vi "replace_file_extension.vi"(8 "error in (no error)":errorcluster, 10 "new_extension":string, 11 "data_path":path) -> (0 "error out":errorcluster, 3 "appended path":path)   [LabVIEW 2018]
panel:
  out "filename without extension":string
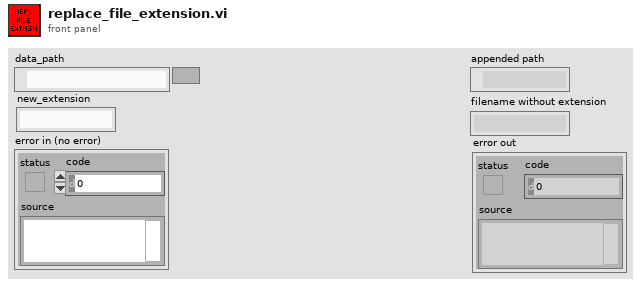
[diagram p1: front panel]
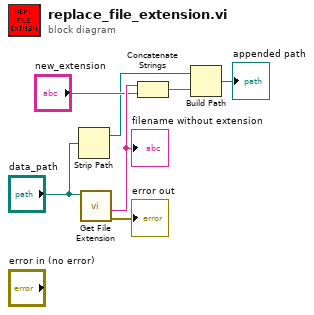
[diagram p0: block diagram]
diagram:
  n1 = Strip Path(path="data_path") -> (stripped path=w4:path)  [unwired: 1 out]
  n2 = call <vilib>:"Get File Extension.vi"("file"="data_path") -> ("error out"=→"error out":errorcluster, "filename without extension"=w7:string)  [unwired: 6 in, 3 out]
  "filename without extension" <- w7
  n3 = Concatenate Strings(w7, "new_extension") -> (w3:string)
  n4 = Build Path(base path=w4, name or relative path=w3) -> (appended path=→"appended path":path)
